vi "OAT Resample Filter Prototype Design.vi"(6 "alias free":bool, 7 "reset? (True)":bool=TRUE, 8 "error in (no error)":errorcluster, 9 "resolution":u16(ring) items=["normal", "high"], 10 "timing jitter":enum32{"Interpolation", "Rounding"}(ring)) -> (0 "error out":errorcluster, 2 "taps":i32, 3 "filter prototype":T1={"left wing"=[], "increment"=[], "max dec"=128, "timing jitter"=enum."Interpolation", "band limiting?"=TRUE} {"increment" format="%.2f"; "left wing" format="%.2f"})   [LabVIEW 2017, in "SoundVib_Resampling.lvlib"]
doc: "Design a filter prototype for arbitrary resampling."
uses:
  <vilib>/addons/Sound and Vibration/Order Analysis/Resample Order Tracking/SoundVib_Resampling.lvlib
  <vilib>/addons/_NISVFA/_Shared subVIs/Controls/OAT Resample Filter Prototype.ctl
panel:
  in  "maximum decimation\nfactor (auto)":i32
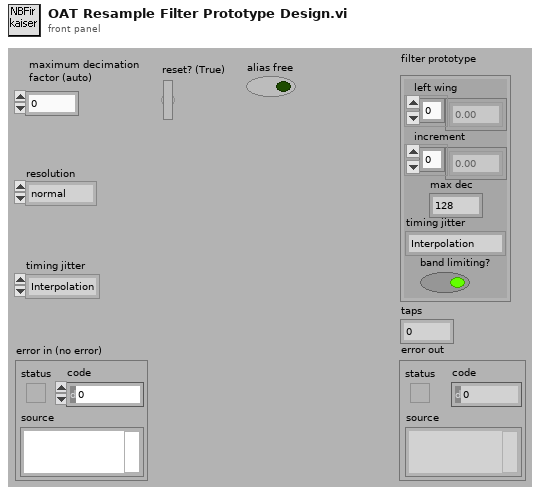
[diagram p1: front panel]
types:
  T1 = typedef "OAT Resample Filter Prototype.ctl" = cluster{"left wing":dbl[], "increment":dbl[], "max dec":i32, "timing jitter":enum32{"Interpolation", "Rounding"}, "band limiting?":bool}
  T2 = cluster{"maximum decimation\nfactor (auto)":i32, "alias free":bool, dbl, "timing jitter":enum32{"Interpolation", "Rounding"}}
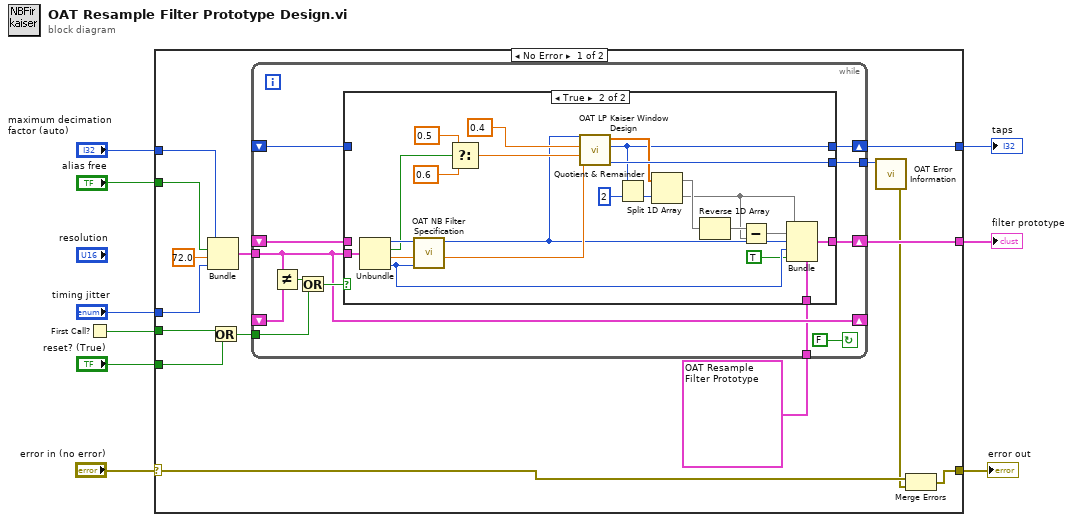
[diagram p0: block diagram]
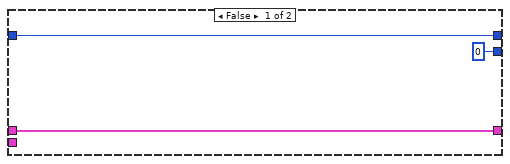
[diagram p2: hidden frame]
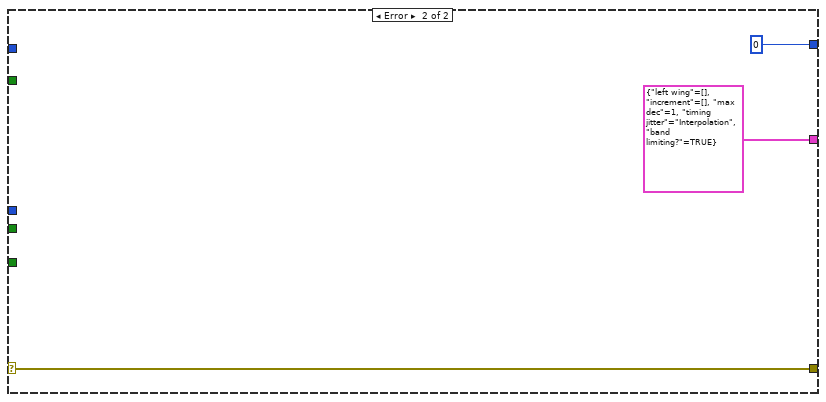
[diagram p3: hidden frame]
diagram:
  n1 = First Call?() -> (First Call?: T/F=w3:bool)
  n2 = case shown="No Error" "error in (no error)" {
    selector: "error in (no error)" -> [w12 w65]
    tunnel: [w24 T1 {"left wing"=[], "increment"=[], "max dec"=1, "timing jitter"=enum."Interpolation", "band limiting?"=TRUE} ("filter prototype")] -> w9
    tunnel: [w22 0 ("taps")] -> w8
    tunnel: "timing jitter" -> [w21 _]
    tunnel: "maximum decimation\nfactor (auto)" -> [w20 _]
    tunnel: "alias free" -> [w19 _]
    tunnel: "reset? (True)" -> [w16 _]
    tunnel: w3 -> [w15 _]
    tunnel: [w10 w65] -> w1
    frame No Error {
      n3 = Bundle("maximum decimation\nfactor (auto)"=w20, "alias free"=w19, 72.0, "timing jitter"=w21) -> (w23:T2)  [unwired: 1 in]
      n4 = Or(x=w15, y=w16) -> (x .or. y?=w14:bool)
      n5 = while {
        shift-right: [w36] -> w24
        shift-left: _ -> [w30]
        shift-right: [w27] -> _
        shift-left: _ -> [w28]
        tunnel: w23 -> [w27]
        shift-right: [w34] -> w22
        shift-left: _ -> [w29]
        tunnel: w14 -> [w33]
        tunnel: [w26] -> w18
        tunnel: T1 {"left wing"=array[915 elements], "increment"=array[914 elements], "max dec"=128, "timing jitter"=enum."Interpolation", "band limiting?"=TRUE} ("filter prototype") -> [w25]
        stop <- FALSE continue-if-true
        n6 = Not Equal?(x=w27, y=w28) -> (x != y?=w32:bool)
        n7 = Or(x=w32, y=w33) -> (x .or. y?=w31:bool)
        n8 = case shown="True" w31 {
          tunnel: [w39 w48] -> w34
          tunnel: [w38 w60] -> w36
          tunnel: w27 -> [_ w59]
          tunnel: w29 -> [w39 _]
          tunnel: w30 -> [w38 _]
          tunnel: [0 ("error") w51] -> w26
          tunnel: w25 -> [_ w44]
          frame False {
          }
          frame True {
            n9 = Unbundle(w59) -> ("maximum decimation\nfactor (auto)"=w56:i32, "alias free"=w53:bool, w55:dbl, "timing jitter"=w43:enum32{"Interpolation", "Rounding"})
            n10 = call <vilib>:"OAT NB Filter Specification.vi"("timing jitter"=w43, "stop band attenuation"=w55, "maximum decimation factor"=w56) -> ("A stop [dB]"=w54:dbl, "decimation factor"=w52:i32)  [unwired: 7 in]
            n11 = Select(t=0.5, s=w53, f=0.6) -> (s? t:f=w57:dbl)
            n12 = call <vilib>:"OAT LP Kaiser Window Design.vi"("A stop [dB]"=w54, "stopband"=w57, "passband"=0.4 ("low cutoff freq: fl"), "fs"=w52) -> ("error"=w51:i32, "taps"=w48:i32, "filter coefficients"=w50:dbl[])  [unwired: 5 in]
            n13 = Quotient & Remainder(x=w48, y=2) -> (floor(x/y)=w49:i32)  [unwired: 1 out]
            n14 = Split 1D Array(array=w50, index=w49) -> (first subarray=w46:dbl[], second subarray=w40:dbl[])
            n15 = Reverse 1D Array(array=w46) -> (reversed array=w41:dbl[])
            n16 = Subtract(x=w41, y=w40) -> (x-y=w45:dbl[])
            n17 = Bundle(cluster=w44, "left wing"=w40, "increment"=w45, "max dec"=w52, "timing jitter"=w43, "band limiting?"=TRUE) -> (w60:T1)
          }
        }
      }
      n18 = call <vilib>:"OAT Error Information.vi"("error code"=w18) -> ("error out"=w11:errorcluster)  [unwired: 6 in]
      n19 = Merge Errors(w12, w11) -> (w10:errorcluster)
    }
    frame Error {
    }
  }
  "filter prototype" <- w9
  "taps" <- w8
  "error out" <- w1
